vi "invatare.vi"() -> ()   [LabVIEW 2024]
uses:
  <vilib>/National Instruments/NI Super Simple Neural Networks/Types/Teaching Settings.ctl
  <vilib>/National Instruments/NI Super Simple Neural Networks/Types/Error Evaluation.ctl
  <vilib>/National Instruments/NI Super Simple Neural Networks/API/Create 2 Hidden Layers.vi
  <vilib>/National Instruments/NI Super Simple Neural Networks/Neural Network.lvclass
panel:
  out "Teaching Time (s)":dbl
  out "Solution Found":bool
  out "Waveform Graph":dbl[](graph)
  out "Error Trend Out":dbl[](array[numeric])
  in  "NN-Config name":path
  in  "Settings In":T1={"Max Epocs"=10000, "Error Goal"=10.0, "Max Time (s)"=10.0, "Error Evaluation"=enum."Over Teaching Set", "# Vectors per Iteration"=200}
  in  "2nd Hidden Layer Neurons":u32
  in  "1st Hidden Layer Neurons":u32
  out "nume clase":string[](array[string])
  in  "NN- Trained file name":path
  in  "Dataset folder":path
  in  "Output Layer Linear (False)":bool
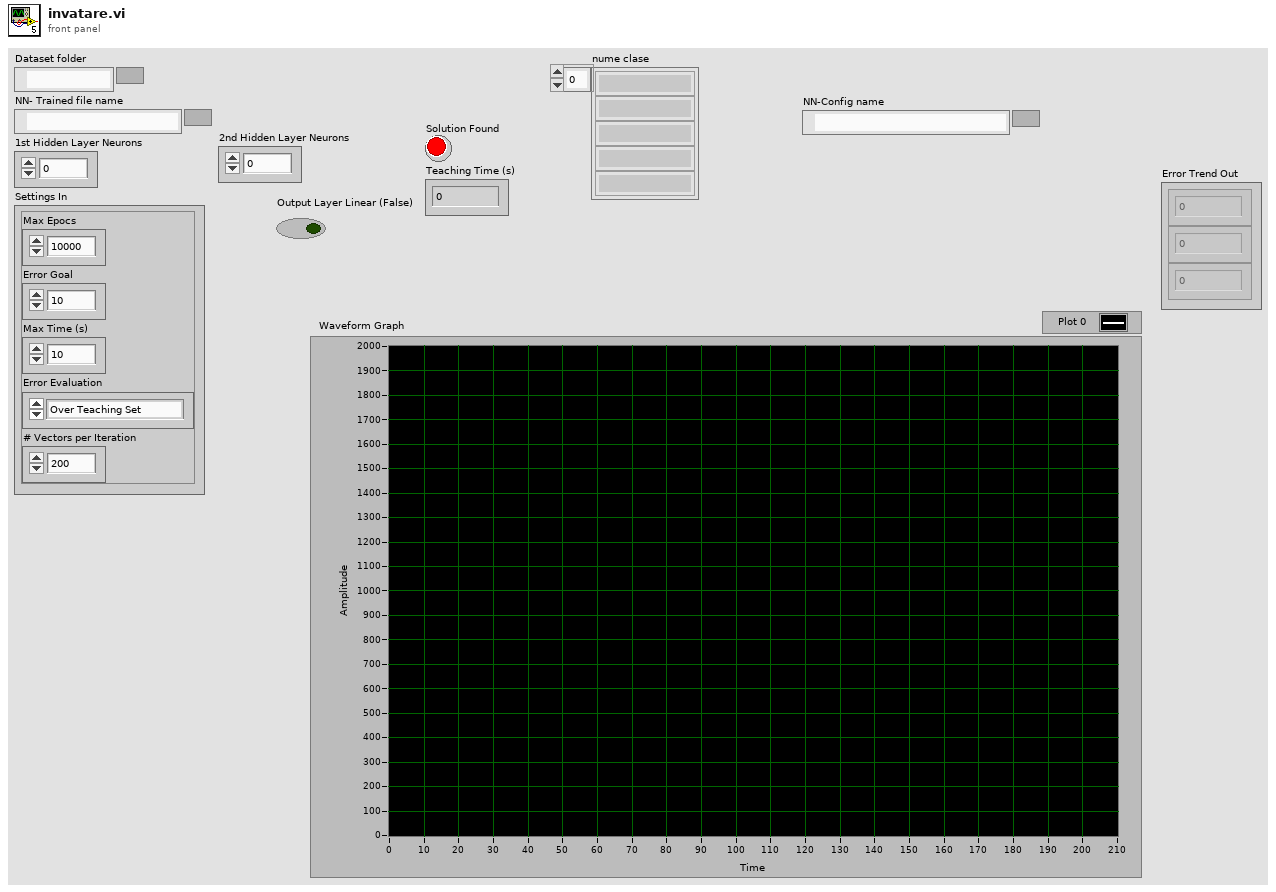
[diagram p1: front panel]
types:
  T1 = typedef "Neural Network.lvclass/Teaching Settings.ctl" = cluster{"Max Epocs":u64, "Error Goal":dbl, "Max Time (s)":dbl, "Error Evaluation":T2, "# Vectors per Iteration":i32}
  T2 = typedef "Neural Network.lvclass/Error Evaluation.ctl" = enum16{"Over Both Sets", "Over Validation Set", "Over Teaching Set"}
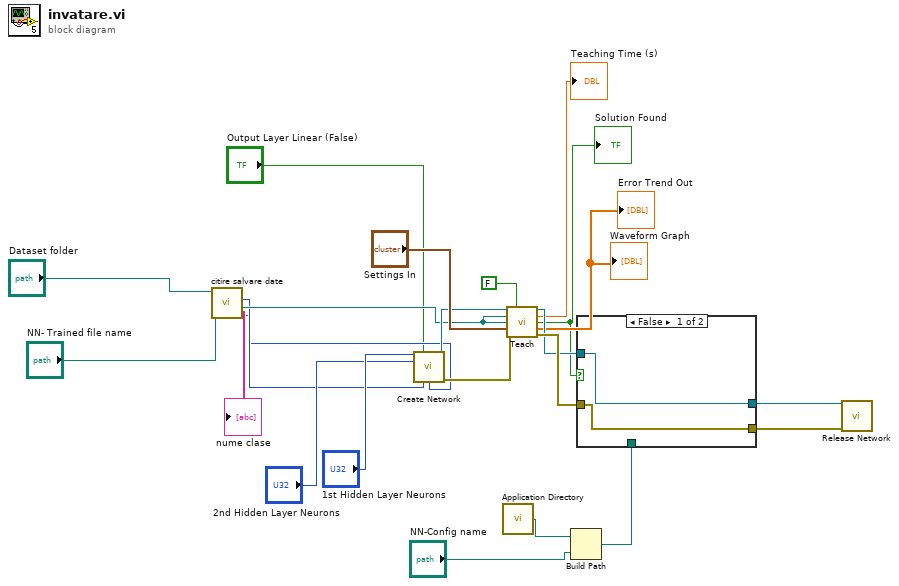
[diagram p0: block diagram]
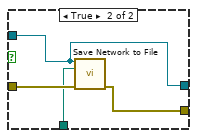
[diagram p2: hidden frame]
diagram:
  n1 = call "citire salvare date.vi"("NN- Trained file name"="NN- Trained file name", "Dataset folder"="Dataset folder") -> ("RN outputs"=w3:i32, "DataSet Trainded data"=w5:path, "Inputs"=w4:i32, "nume clase"=→"nume clase":string[])  [unwired: 5 in, 1 out]
  n2 = call-poly <vilib>:"Create Network.vi"("1st Hidden Layer Neurons"="1st Hidden Layer Neurons", "Output Layer Linear (False)"="Output Layer Linear (False)", "2nd Hidden Layer Neurons"="2nd Hidden Layer Neurons", "# Inputs"=w4, "Output Neurons/Outputs"=w3) -> ("Neural Network"=w6:refnum<class "Neural Network.lvclass">, "Error Out"=w16:errorcluster)  [unwired: 9 in]
  n3 = call <vilib>:"Application Directory.vi"() -> ("Application Directory"=w14:path)
  n4 = call <vilib>:"Teach.vi"("Neural Network In"=w6, "Enable Growing/Prunning"=FALSE, "Teaching Set Path In"=w5, "Validation Set Path In"=w5, "Settings In"="Settings In", "Error In"=w16) -> ("Neural Network Out"=w11:refnum<class "Neural Network.lvclass">, "Teaching Time (s)"=→"Teaching Time (s)":dbl, "Solution Found"=w7:bool, "Error Trend Out"=→"Error Trend Out" →"Waveform Graph":dbl[], "Error Out"=w15:errorcluster)  [unwired: 5 in]
  "Solution Found" <- w7
  n5 = Build Path(base path=w14, name or relative path="NN-Config name") -> (appended path=w12:path)
  n6 = case shown="False" w7 {
    tunnel: w11 -> [w24 w26]
    tunnel: w15 -> [w25 w29]
    tunnel: w12 -> [_ w28]
    tunnel: [w25 w27] -> w10
    tunnel: [w24 w26] -> w1
    frame False {
    }
    frame True {
      n7 = call <vilib>:"Save Network to File.vi"("Neural Network In"=w26, "File Path (dialog)"=w28, "Error In"=w29) -> ("Error Out"=w27:errorcluster)  [unwired: 10 in, 2 out]
    }
  }
  n8 = call <vilib>:"Release Network.vi"("Neural Network"=w1, "Error In"=w10) -> ()  [unwired: 13 in, 1 out]
